vi "rsidr_core_global.vi"() -> ()   [LabVIEW 2015, in "Rohde&Schwarz CMXP GPRF.lvlib"]
doc: "This Global variable contains driver's:\n- Attributes\n- Range Tables\n- Repeated Capabilities"
uses:
  <instrlib>/Rohde&Schwarz CMXP GPRF/Rohde&Schwarz CMXP GPRF.lvlib
  <instrlib>/Rohde&Schwarz CMXP GPRF/Private/rsidr_core.llb/type_Input_Format_Attribute.ctl
  <instrlib>/Rohde&Schwarz CMXP GPRF/Private/rsidr_core.llb/type_Input_Format_RangeTable.ctl
  <instrlib>/Rohde&Schwarz CMXP GPRF/Private/rsidr_core.llb/type_Input_Format_RepCap.ctl
  <instrlib>/Rohde&Schwarz CMXP GPRF/Private/rsidr_core.llb/rsidr_core.lvlib
panel:
  in  "Repeated Capabilities":T1[](array[typedef])
  in  "Range Tables":T2[](array[typedef])=[{"Type"=2, "Name"="rsCmxpGprf_rngInputConnector", "Entries"=[{"Name"="RF 1 COM", "Value 1"=1.0, "Value 2"=0.0, "Command"="RF1C"}, {"Name"="RF 2 COM", "Value 1"=2.0, "Value 2"=0.0, "Command"="RF2C"}, {"Name"="RF 2 IN", "Value 1"=3.0, "Value 2"=0.0, "Command"="RF2I"}, {"Name"="RF 3 COM", "Value 1"=4.0, "Value 2"=0.0, "Command"="RF3C"}, {"Name"="RF 4 COM", "Value 1"=5.0, "Value 2"=0.0, "Command"="RF4C"}, {"Name"="RF 4 IN", "Value 1"=6.0, "Value 2"=0.0, "Command"="RF4I"}, {"Name"="IQ 1 IN", "Value 1"=7.0, "Value 2"=0.0, "Command"="IQ1I"}, {"Name"="IQ 3 IN", "Value 1"=8.0, "Value 2"=0.0, "Command"="IQ3I"}, {"Name"="IQ 5 IN", "Value 1"=9.0, "Value 2"=0.0, "Command"="IQ5I"}, {"Name"="IQ 7 IN", "Value 1"=10.0, "Value 2"=0.0, "Command"="IQ7I"}, {"Name"="RF 11", "Value 1"=11.0, "Value 2"=0.0, "Command"="R11"}, {"Name"="RF 12", "Value 1"=12.0, "Value 2"=0.0, "Command"="R12"}, {"Name"="RF 13", "Value 1"=13.0, "Value 2"=0.0, "Command"="R13"}, {"Name"="RF 14", "Value 1"=14.0, "Value 2"=0.0, "Command"="R14"}, {"Name"="RF 15", "Value 1"=15.0, "Value 2"=0.0, "Command"="R15"}, {"Name"="RF 16", "Value 1"=16.0, "Value 2"=0.0, "Command"="R16"}, {"Name"="RF 17", "Value 1"=17.0, "Value 2"=0.0, "Command"="R17"}, {"Name"="RF 18", "Value 1"=18.0, "Value 2"=0.0, "Command"="R18"}, {"Name"="RF 21", "Value 1"=19.0, "Value 2"=0.0, "Command"="R21"}, {"Name"="RF 22", "Value 1"=20.0, "Value 2"=0.0, "Command"="R22"}, {"Name"="RF 23", "Value 1"=21.0, "Value 2"=0.0, "Command"="R23"}, {"Name"="RF 24", "Value 1"=22.0, "Value 2"=0.0, "Command"="R24"}, {"Name"="RF 25", "Value 1"=23.0, "Value 2"=0.0, "Command"="R25"}, {"Name"="RF 26", "Value 1"=24.0, "Value 2"=0.0, "Command"="R26"}, {"Name"="RF 27", "Value 1"=25.0, "Value 2"=0.0, "Command"="R27"}, {"Name"="RF 28", "Value 1"=26.0, "Value 2"=0.0, "Command"="R28"}, {"Name"="RF 31", "Value 1"=27.0, "Value 2"=0.0, "Command"="R31"}, {"Name"="RF 32", "Value 1"=28.0, "Value 2"=0.0, "Command"="R32"}, {"Name"="RF 33", "Value 1"=29.0, "Value 2"=0.0, "Command"="R33"}, {"Name"="RF 34", "Value 1"=30.0, "Value 2"=0.0, "Command"="R34"}, {"Name"="RF 35", "Value 1"=31.0, "Value 2"=0.0, "Command"="R35"}, {"Name"="RF 36", "Value 1"=32.0, "Value 2"=0.0, "Command"="R36"}, {"Name"="RF 37", "Value 1"=33.0, "Value 2"=0.0, "Command"="R37"}, {"Name"="RF 38", "Value 1"=34.0, "Value 2"=0.0, "Command"="R38"}, {"Name"="RF 41", "Value 1"=35.0, "Value 2"=0.0, "Command"="R41"}, {"Name"="RF 42", "Value 1"=36.0, "Value 2"=0.0, "Command"="R42"}, {"Name"="RF 43", "Value 1"=37.0, "Value 2"=0.0, "Command"="R43"}, {"Name"="RF 44", "Value 1"=38.0, "Value 2"=0.0, "Command"="R44"}, {"Name"="RF 45", "Value 1"=39.0, "Value 2"=0.0, "Command"="R45"}, {"Name"="RF 46", "Value 1"=40.0, "Value 2"=0.0, "Command"="R46"}, {"Name"="RF 47", "Value 1"=41.0, "Value 2"=0.0, "Command"="R47"}, {"Name"="RF 48", "Value 1"=42.0, "Value 2"=0.0, "Command"="R48"}, {"Name"="RF 11 COM", "Value 1"=43.0, "Value 2"=0.0, "Command"="R11C"}, {"Name"="RF 12 COM", "Value 1"=44.0, "Value 2"=0.0, "Command"="R12C"}, {"Name"="RF 12 IN", "Value 1"=45.0, "Value 2"=0.0, "Command"="R12I"}, {"Name"="RF 13 COM", "Value 1"=46.0, "Value 2"=0.0, "Command"="R13C"}, {"Name"="RF 14 COM", "Value 1"=47.0, "Value 2"=0.0, "Command"="R14C"}, {"Name"="RF 14 IN", "Value 1"=48.0, "Value 2"=0.0, "Command"="R14I"}, {"Name"="IQ 11 IN", "Value 1"=49.0, "Value 2"=0.0, "Command"="I11I"}, {"Name"="IQ 13 IN", "Value 1"=50.0, "Value 2"=0.0, "Command"="I13I"}, {"Name"="IQ 15 IN", "Value 1"=51.0, "Value 2"=0.0, "Command"="I15I"}, {"Name"="IQ 17 IN", "Value 1"=52.0, "Value 2"=0.0, "Command"="I17I"}, {"Name"="RF 21 COM", "Value 1"=53.0, "Value 2"=0.0, "Command"="R21C"}, {"Name"="RF 22 COM", "Value 1"=54.0, "Value 2"=0.0, "Command"="R22C"}, {"Name"="RF 22 IN", "Value 1"=55.0, "Value 2"=0.0, "Command"="R22I"}, {"Name"="RF 23 COM", "Value 1"=56.0, "Value 2"=0.0, "Command"="R23C"}, {"Name"="RF 24 COM", "Value 1"=57.0, "Value 2"=0.0, "Command"="R24C"}, {"Name"="RF 24 IN", "Value 1"=58.0, "Value 2"=0.0, "Command"="R24I"}, {"Name"="IQ 21 IN", "Value 1"=59.0, "Value 2"=0.0, "Command"="I21I"}, {"Name"="IQ 23 IN", "Value 1"=60.0, "Value 2"=0.0, "Command"="I23I"}, {"Name"="IQ 25 IN", "Value 1"=61.0, "Value 2"=0.0, "Command"="I25I"}, {"Name"="IQ 27 IN", "Value 1"=62.0, "Value 2"=0.0, "Command"="I27I"}, {"Name"="RF 31 COM", "Value 1"=63.0, "Value 2"=0.0, "Command"="R31C"}, {"Name"="RF 32 COM", "Value 1"=64.0, "Value 2"=0.0, "Command"="R32C"}, {"Name"="RF 32 IN", "Value 1"=65.0, "Value 2"=0.0, "Command"="R32I"}, {"Name"="RF 33 COM", "Value 1"=66.0, "Value 2"=0.0, "Command"="R33C"}, {"Name"="RF 34 COM", "Value 1"=67.0, "Value 2"=0.0, "Command"="R34C"}, {"Name"="RF 34 IN", "Value 1"=68.0, "Value 2"=0.0, "Command"="R34I"}, {"Name"="IQ 31 IN", "Value 1"=69.0, "Value 2"=0.0, "Command"="I31I"}, {"Name"="IQ 33 IN", "Value 1"=70.0, "Value 2"=0.0, "Command"="I33I"}, {"Name"="IQ 35 IN", "Value 1"=71.0, "Value 2"=0.0, "Command"="I35I"}, {"Name"="IQ 37 IN", "Value 1"=72.0, "Value 2"=0.0, "Command"="I37I"}, {"Name"="RF 41 COM", "Value 1"=73.0, "Value 2"=0.0, "Command"="R41C"}, {"Name"="RF 42 COM", "Value 1"=74.0, "Value 2"=0.0, "Command"="R42C"}, {"Name"="RF 42 IN", "Value 1"=75.0, "Value 2"=0.0, "Command"="R42I"}, {"Name"="RF 43 COM", "Value 1"=76.0, "Value 2"=0.0, "Command"="R43C"}, {"Name"="RF 44 COM", "Value 1"=77.0, "Value 2"=0.0, "Command"="R44C"}, {"Name"="RF 44 IN", "Value 1"=78.0, "Value 2"=0.0, "Command"="R44I"}, {"Name"="IQ 41 IN", "Value 1"=79.0, "Value 2"=0.0, "Command"="I41I"}, {"Name"="IQ 43 IN", "Value 1"=80.0, "Value 2"=0.0, "Command"="I43I"}, {"Name"="IQ 45 IN", "Value 1"=81.0, "Value 2"=0.0, "Command"="I45I"}, {"Name"="IQ 47 IN", "Value 1"=82.0, "Value 2"=0.0, "Command"="I47I"}, {"Name"="RF A COM", "Value 1"=83.0, "Value 2"=0.0, "Command"="RFAC"}, {"Name"="RF B COM", "Value 1"=84.0, "Value 2"=0.0, "Command"="RFBC"}, {"Name"="RF B IN", "Value 1"=85.0, "Value 2"=0.0, "Command"="RFBI"}, {"Name"="RF A 1", "Value 1"=86.0, "Value 2"=0.0, "Command"="RA1"}, {"Name"="RF A 2", "Value 1"=87.0, "Value 2"=0.0, "Command"="RA2"}, {"Name"="RF A 3", "Value 1"=88.0, "Value 2"=0.0, "Command"="RA3"}, {"Name"="RF A 4", "Value 1"=89.0, "Value 2"=0.0, "Command"="RA4"}, {"Name"="RF A 5", "Value 1"=90.0, "Value 2"=0.0, "Command"="RA5"}, {"Name"="RF A 6", "Value 1"=91.0, "Value 2"=0.0, "Command"="RA6"}, {"Name"="RF A 7", "Value 1"=92.0, "Value 2"=0.0, "Command"="RA7"}, {"Name"="RF A 8", "Value 1"=93.0, "Value 2"=0.0, "Command"="RA8"}, {"Name"="RF B 1", "Value 1"=94.0, "Value 2"=0.0, "Command"="RB1"}, {"Name"="RF B 2", "Value 1"=95.0, "Value 2"=0.0, "Command"="RB2"}, {"Name"="RF B 3", "Value 1"=96.0, "Value 2"=0.0, "Command"="RB3"}, {"Name"="RF B 4", "Value 1"=97.0, "Value 2"=0.0, "Command"="RB4"}, {"Name"="RF B 5", "Value 1"=98.0, "Value 2"=0.0, "Command"="RB5"}, {"Name"="RF B 6", "Value 1"=99.0, "Value 2"=0.0, "Command"="RB6"}, {"Name"="RF B 7", "Value 1"=100.0, "Value 2"=0.0, "Command"="RB7"}, {"Name"="RF B 8", "Value 1"=101.0, "Value 2"=0.0, "Command"="RB8"}]}, {"Type"=0, "Name"="rsCmxpGprf_rngExtAtt", "Entries"=[{"Name"="", "Value 1"=-50.0, "Value 2"=90.0, "Command"=""}]}, {"Type"=0, "Name"="rsCmxpGprf_rngCenterFrequency", "Entries"=[{"Name"="", "Value 1"=70000000.0, "Value 2"=6000000000.0, "Command"=""}]}, {"Type"=2, "Name"="rsCmxpGprf_rngOutputConnector", "Entries"=[{"Name"="RF 1 OUT", "Value 1"=0.0, "Value 2"=0.0, "Command"="RF1O"}, {"Name"="RF 1 COM", "Value 1"=1.0, "Value 2"=0.0, "Command"="RF1C"}, {"Name"="RF 2 COM", "Value 1"=2.0, "Value 2"=0.0, "Command"="RF2C"}, {"Name"="RF 3 COM", "Value 1"=3.0, "Value 2"=0.0, "Command"="RF3C"}, {"Name"="RF 3 OUT", "Value 1"=4.0, "Value 2"=0.0, "Command"="RF3O"}, {"Name"="RF 4 COM", "Value 1"=5.0, "Value 2"=0.0, "Command"="RF4C"}, {"Name"="IQ 2 OUT", "Value 1"=6.0, "Value 2"=0.0, "Command"="IQ2O"}, {"Name"="IQ 4 OUT", "Value 1"=7.0, "Value 2"=0.0, "Command"="IQ4O"}, {"Name"="IQ 6 OUT", "Value 1"=8.0, "Value 2"=0.0, "Command"="IQ6O"}, {"Name"="IQ 8 OUT", "Value 1"=9.0, "Value 2"=0.0, "Command"="IQ8O"}, {"Name"="RF 118", "Value 1"=10.0, "Value 2"=0.0, "Command"="R118"}, {"Name"="RF 218", "Value 1"=11.0, "Value 2"=0.0, "Command"="R218"}, {"Name"="RF 214", "Value 1"=12.0, "Value 2"=0.0, "Command"="R214"}, {"Name"="RF 258", "Value 1"=13.0, "Value 2"=0.0, "Command"="R258"}, {"Name"="RF 318", "Value 1"=14.0, "Value 2"=0.0, "Command"="R318"}, {"Name"="RF 418", "Value 1"=15.0, "Value 2"=0.0, "Command"="R418"}, {"Name"="RF 11 COM", "Value 1"=16.0, "Value 2"=0.0, "Command"="R11C"}, {"Name"="RF 11 OUT", "Value 1"=17.0, "Value 2"=0.0, "Command"="R11O"}, {"Name"="RF 12 COM", "Value 1"=18.0, "Value 2"=0.0, "Command"="R12C"}, {"Name"="RF 13 COM", "Value 1"=19.0, "Value 2"=0.0, "Command"="R13C"}, {"Name"="RF 13 OUT", "Value 1"=20.0, "Value 2"=0.0, "Command"="R13O"}, {"Name"="RF 14 COM", "Value 1"=21.0, "Value 2"=0.0, "Command"="R14C"}, {"Name"="IQ 12 OUT", "Value 1"=22.0, "Value 2"=0.0, "Command"="I12O"}, {"Name"="IQ 14 OUT", "Value 1"=23.0, "Value 2"=0.0, "Command"="I14O"}, {"Name"="IQ 16 OUT", "Value 1"=24.0, "Value 2"=0.0, "Command"="I16O"}, {"Name"="IQ 18 OUT", "Value 1"=25.0, "Value 2"=0.0, "Command"="I18O"}, {"Name"="RF 21 COM", "Value 1"=26.0, "Value 2"=0.0, "Command"="R21C"}, {"Name"="RF 21 OUT", "Value 1"=27.0, "Value 2"=0.0, "Command"="R21O"}, {"Name"="RF 22 COM", "Value 1"=28.0, "Value 2"=0.0, "Command"="R22C"}, {"Name"="RF 23 COM", "Value 1"=29.0, "Value 2"=0.0, "Command"="R23C"}, {"Name"="RF 23 OUT", "Value 1"=30.0, "Value 2"=0.0, "Command"="R23O"}, {"Name"="RF 24 COM", "Value 1"=31.0, "Value 2"=0.0, "Command"="R24C"}, {"Name"="IQ 22 OUT", "Value 1"=32.0, "Value 2"=0.0, "Command"="I22O"}, {"Name"="IQ 24 OUT", "Value 1"=33.0, "Value 2"=0.0, "Command"="I24O"}, {"Name"="IQ 26 OUT", "Value 1"=34.0, "Value 2"=0.0, "Command"="I26O"}, {"Name"="IQ 28 OUT", "Value 1"=35.0, "Value 2"=0.0, "Command"="I28O"}, {"Name"="RF 31 COM", "Value 1"=36.0, "Value 2"=0.0, "Command"="R31C"}, {"Name"="RF 31 OUT", "Value 1"=37.0, "Value 2"=0.0, "Command"="R31O"}, {"Name"="RF 32 COM", "Value 1"=38.0, "Value 2"=0.0, "Command"="R32C"}, {"Name"="RF 33 COM", "Value 1"=39.0, "Value 2"=0.0, "Command"="R33C"}, {"Name"="RF 33 OUT", "Value 1"=40.0, "Value 2"=0.0, "Command"="R33O"}, {"Name"="RF 34 COM", "Value 1"=41.0, "Value 2"=0.0, "Command"="R34C"}, {"Name"="IQ 32 OUT", "Value 1"=42.0, "Value 2"=0.0, "Command"="I32O"}, {"Name"="IQ 34 OUT", "Value 1"=43.0, "Value 2"=0.0, "Command"="I34O"}, {"Name"="IQ 36 OUT", "Value 1"=44.0, "Value 2"=0.0, "Command"="I36O"}, {"Name"="IQ 38 OUT", "Value 1"=45.0, "Value 2"=0.0, "Command"="I38O"}, {"Name"="RF 41 COM", "Value 1"=46.0, "Value 2"=0.0, "Command"="R41C"}, {"Name"="RF 41 OUT", "Value 1"=47.0, "Value 2"=0.0, "Command"="R41O"}, {"Name"="RF 42 COM", "Value 1"=48.0, "Value 2"=0.0, "Command"="R42C"}, {"Name"="RF 43 COM", "Value 1"=49.0, "Value 2"=0.0, "Command"="R43C"}, {"Name"="RF 43 OUT", "Value 1"=50.0, "Value 2"=0.0, "Command"="R43O"}, {"Name"="RF 44 COM", "Value 1"=51.0, "Value 2"=0.0, "Command"="R44C"}, {"Name"="IQ 42 OUT", "Value 1"=52.0, "Value 2"=0.0, "Command"="I42O"}, {"Name"="IQ 44 OUT", "Value 1"=53.0, "Value 2"=0.0, "Command"="I44O"}, {"Name"="IQ 46 OUT", "Value 1"=54.0, "Value 2"=0.0, "Command"="I46O"}, {"Name"="IQ 48 OUT", "Value 1"=55.0, "Value 2"=0.0, "Command"="I48O"}, {"Name"="RF A COM", "Value 1"=56.0, "Value 2"=0.0, "Command"="RFAC"}, {"Name"="RF A OUT", "Value 1"=57.0, "Value 2"=0.0, "Command"="RFAO"}, {"Name"="RF B COM", "Value 1"=58.0, "Value 2"=0.0, "Command"="RFBC"}, {"Name"="RF A 18", "Value 1"=59.0, "Value 2"=0.0, "Command"="RA18"}, {"Name"="RF B 14", "Value 1"=60.0, "Value 2"=0.0, "Command"="RB14"}, {"Name"="RF B 18", "Value 1"=61.0, "Value 2"=0.0, "Command"="RB18"}]}, {"Type"=0, "Name"="rsCmxpGprf_rngGeneratorLevel", "Entries"=[{"Name"="", "Value 1"=-130.0, "Value 2"=0.0, "Command"=""}]}, {"Type"=2, "Name"="rsCmxpGprf_rngBasebandMode", "Entries"=[{"Name"="CW", "Value 1"=0.0, "Value 2"=0.0, "Command"="CW"}, {"Name"="Dual Tone", "Value 1"=1.0, "Value 2"=0.0, "Command"="DTON"}, {"Name"="ARB", "Value 1"=2.0, "Value 2"=0.0, "Command"="ARB"}]}, {"Type"=0, "Name"="rsCmxpGprf_rngDtoneFrequency", "Entries"=[{"Name"="", "Value 1"=-40000000.0, "Value 2"=40000000.0, "Command"=""}]}, {"Type"=0, "Name"="rsCmxpGprf_rngDtoneRatio", "Entries"=[{"Name"="", "Value 1"=0.0, "Value 2"=30.0, "Command"=""}]}, {"Type"=0, "Name"="rsCmxpGprf_rngListModeDwellTime", "Entries"=[{"Name"="", "Value 1"=0.0002, "Value 2"=20.0, "Command"=""}]}, {"Type"=0, "Name"="rsCmxpGprf_rngListLevel", "Entries"=[{"Name"="", "Value 1"=-130.0, "Value 2"=13.0, "Command"=""}]}, {"Type"=0, "Name"="rsCmxpGprf_rngDigitalGain", "Entries"=[{"Name"="", "Value 1"=-30.0, "Value 2"=0.0, "Command"=""}]}, {"Type"=0, "Name"="rsCmxpGprf_rngStepLength", "Entries"=[{"Name"="", "Value 1"=5e-05, "Value 2"=1.0, "Command"=""}]}, {"Type"=0, "Name"="rsCmxpGprf_rngMeasLength", "Entries"=[{"Name"="", "Value 1"=5e-05, "Value 2"=0.0003, "Command"=""}]}, {"Type"=2, "Name"="rsCmxpGprf_rngRepMode", "Entries"=[{"Name"="Single", "Value 1"=0.0, "Value 2"=0.0, "Command"="SING"}, {"Name"="Continuous", "Value 1"=1.0, "Value 2"=0.0, "Command"="CONT"}]}, {"Type"=0, "Name"="rsCmxpGprf_rngStatCount", "Entries"=[{"Name"="", "Value 1"=1.0, "Value 2"=1000.0, "Command"=""}]}, {"Type"=2, "Name"="rsCmxpGprf_rngPowerMeasFilterType", "Entries"=[{"Name"="Gauss", "Value 1"=0.0, "Value 2"=0.0, "Command"="GAUS"}, {"Name"="Bandpass", "Value 1"=1.0, "Value 2"=0.0, "Command"="BAND"}, {"Name"="WCDMA", "Value 1"=2.0, "Value 2"=0.0, "Command"="WCDM"}, {"Name"="CDMA", "Value 1"=3.0, "Value 2"=0.0, "Command"="CDMA"}, {"Name"="TD-SCDMA", "Value 1"=4.0, "Value 2"=0.0, "Command"="TDSC"}]}, {"Type"=1, "Name"="rsCmxpGprf_rngGaussBwid", "Entries"=[{"Name"="", "Value 1"=1000.0, "Value 2"=0.0, "Command"=""}, {"Name"="", "Value 1"=10000.0, "Value 2"=0.0, "Command"=""}, {"Name"="", "Value 1"=100000.0, "Value 2"=0.0, "Command"=""}, {"Name"="", "Value 1"=1000000.0, "Value 2"=0.0, "Command"=""}, {"Name"="", "Value 1"=10000000.0, "Value 2"=0.0, "Command"=""}]}, {"Type"=1, "Name"="rsCmxpGprf_rngBandBwid", "Entries"=[{"Name"="", "Value 1"=1000.0, "Value 2"=0.0, "Command"=""}, {"Name"="", "Value 1"=10000.0, "Value 2"=0.0, "Command"=""}, {"Name"="", "Value 1"=100000.0, "Value 2"=0.0, "Command"=""}, {"Name"="", "Value 1"=1000000.0, "Value 2"=0.0, "Command"=""}, {"Name"="", "Value 1"=10000000.0, "Value 2"=0.0, "Command"=""}, {"Name"="", "Value 1"=40000000.0, "Value 2"=0.0, "Command"=""}, {"Name"="", "Value 1"=160000000.0, "Value 2"=0.0, "Command"=""}]}, {"Type"=2, "Name"="rsCmxpGprf_rngTrigSlope", "Entries"=[{"Name"="Rising", "Value 1"=0.0, "Value 2"=0.0, "Command"="REDG"}, {"Name"="Falling", "Value 1"=1.0, "Value 2"=0.0, "Command"="FEDG"}]}, {"Type"=0, "Name"="rsCmxpGprf_rngTrigThreshold", "Entries"=[{"Name"="", "Value 1"=-50.0, "Value 2"=0.0, "Command"=""}]}, {"Type"=0, "Name"="rsCmxpGprf_rngTrigOffset", "Entries"=[{"Name"="", "Value 1"=-0.15, "Value 2"=0.15, "Command"=""}]}, {"Type"=0, "Name"="rsCmxpGprf_rngTrigTout", "Entries"=[{"Name"="", "Value 1"=0.01, "Value 2"=300.0, "Command"=""}]}, {"Type"=2, "Name"="rsCmxpGprf_rngTrigMode", "Entries"=[{"Name"="Trigger Once", "Value 1"=0.0, "Value 2"=0.0, "Command"="ONCE"}, {"Name"="Retrigger Sweep", "Value 1"=1.0, "Value 2"=0.0, "Command"="SWE"}, {"Name"="Retrigger All", "Value 1"=2.0, "Value 2"=0.0, "Command"="ALL"}, {"Name"="Preselect", "Value 1"=3.0, "Value 2"=0.0, "Command"="PRES"}]}, {"Type"=0, "Name"="rsCmxpGprf_rngPwrListIndex", "Entries"=[{"Name"="", "Value 1"=0.0, "Value 2"=3999.0, "Command"=""}]}, {"Type"=2, "Name"="rsCmxpGprf_rngResolution", "Entries"=[{"Name"="1 dB", "Value 1"=0.0, "Value 2"=0.0, "Command"="PD0"}, {"Name"="0.1 dB", "Value 1"=1.0, "Value 2"=0.0, "Command"="PD1"}, {"Name"="0.01 dB", "Value 1"=2.0, "Value 2"=0.0, "Command"="PD2"}, {"Name"="0.001 dB", "Value 1"=3.0, "Value 2"=0.0, "Command"="PD3"}]}, {"Type"=0, "Name"="rsCmxpGprf_rngExtSensorAttenuation", "Entries"=[{"Name"="", "Value 1"=-50.0, "Value 2"=50.0, "Command"=""}]}, {"Type"=0, "Name"="rsCmxpGprf_rngIqvsStepLength", "Entries"=[{"Name"="", "Value 1"=5e-05, "Value 2"=0.005, "Command"=""}]}, {"Type"=0, "Name"="rsCmxpGprf_rngIqvsMeasLength", "Entries"=[{"Name"="", "Value 1"=1e-05, "Value 2"=0.001, "Command"=""}]}, {"Type"=0, "Name"="rsCmxpGprf_rngIqvsFELimit", "Entries"=[{"Name"="", "Value 1"=-100.0, "Value 2"=-30.0, "Command"=""}]}, {"Type"=0, "Name"="rsCmxpGprf_rngIqvsCount", "Entries"=[{"Name"="", "Value 1"=1.0, "Value 2"=3000.0, "Command"=""}]}, {"Type"=2, "Name"="rsCmxpGprf_rngIqvsFilterType", "Entries"=[{"Name"="Gauss", "Value 1"=0.0, "Value 2"=0.0, "Command"="GAUS"}, {"Name"="Bandpass 1MHz", "Value 1"=1.0, "Value 2"=0.0, "Command"="B1MH"}, {"Name"="Nyquist 1MHz", "Value 1"=2.0, "Value 2"=0.0, "Command"="NY1M"}, {"Name"="Bandpass 10MHz", "Value 1"=3.0, "Value 2"=0.0, "Command"="B10M"}, {"Name"="Nyquist 100kHz", "Value 1"=4.0, "Value 2"=0.0, "Command"="NYQ"}]}, {"Type"=0, "Name"="rsCmxpGprf_rngTriggerGap", "Entries"=[{"Name"="", "Value 1"=0.0, "Value 2"=0.01, "Command"=""}]}, {"Type"=0, "Name"="rsCmxpGprf_rngIqvsListIndex", "Entries"=[{"Name"="", "Value 1"=0.0, "Value 2"=149.0, "Command"=""}]}, {"Type"=2, "Name"="rsCmxpGprf_rngIqRFilterType", "Entries"=[{"Name"="Gauss", "Value 1"=0.0, "Value 2"=0.0, "Command"="GAUS"}, {"Name"="Bandpass", "Value 1"=1.0, "Value 2"=0.0, "Command"="BAND"}]}, {"Type"=1, "Name"="rsCmxpGprf_rngFFTFrequencySpan", "Entries"=[{"Name"="", "Value 1"=1250000.0, "Value 2"=0.0, "Command"=""}, {"Name"="", "Value 1"=2500000.0, "Value 2"=0.0, "Command"=""}, {"Name"="", "Value 1"=5000000.0, "Value 2"=0.0, "Command"=""}, {"Name"="", "Value 1"=10000000.0, "Value 2"=0.0, "Command"=""}, {"Name"="", "Value 1"=20000000.0, "Value 2"=0.0, "Command"=""}, {"Name"="", "Value 1"=40000000.0, "Value 2"=0.0, "Command"=""}]}, {"Type"=1, "Name"="rsCmxpGprf_rngFFTLength", "Entries"=[{"Name"="", "Value 1"=1024.0, "Value 2"=0.0, "Command"=""}, {"Name"="", "Value 1"=2048.0, "Value 2"=0.0, "Command"=""}, {"Name"="", "Value 1"=4096.0, "Value 2"=0.0, "Command"=""}, {"Name"="", "Value 1"=8192.0, "Value 2"=0.0, "Command"=""}, {"Name"="", "Value 1"=16384.0, "Value 2"=0.0, "Command"=""}]}, {"Type"=2, "Name"="rsCmxpGprf_rngFFTDetector", "Entries"=[{"Name"="Peak", "Value 1"=0.0, "Value 2"=0.0, "Command"="PEAK"}, {"Name"="RMS", "Value 1"=1.0, "Value 2"=0.0, "Command"="RMS"}]}, {"Type"=0, "Name"="rsCmxpGprf_rngARBCycles", "Entries"=[{"Name"="", "Value 1"=1.0, "Value 2"=10000.0, "Command"=""}]}, {"Type"=2, "Name"="rsCmxpGprf_rngARBMultisegmentTriggerMode", "Entries"=[{"Name"="Seamless", "Value 1"=0.0, "Value 2"=0.0, "Command"="CSE"}, {"Name"="Continuous", "Value 1"=1.0, "Value 2"=0.0, "Command"="CONT"}, {"Name"="Auto", "Value 1"=2.0, "Value 2"=0.0, "Command"="AUTO"}]}, {"Type"=0, "Name"="rsCmxpGprf_rngIndex", "Entries"=[{"Name"="", "Value 1"=0.0, "Value 2"=1999.0, "Command"=""}]}, {"Type"=0, "Name"="rsCmxpGprf_rngIQvsSlotRatio", "Entries"=[{"Name"="", "Value 1"=0.1, "Value 2"=1.0, "Command"=""}]}, {"Type"=0, "Name"="rsCmxpGprf_rngPeakSearchMarkers", "Entries"=[{"Name"="", "Value 1"=0.0, "Value 2"=5.0, "Command"=""}]}, {"Type"=2, "Name"="rsCmxpGprf_rngLinLog", "Entries"=[{"Name"="Linear", "Value 1"=0.0, "Value 2"=0.0, "Command"="LIN"}, {"Name"="Logarithmic", "Value 1"=1.0, "Value 2"=0.0, "Command"="LOG"}]}, {"Type"=2, "Name"="rsCmxpGprf_rngScenario", "Entries"=[{"Name"="Standalone", "Value 1"=0.0, "Value 2"=0.0, "Command"="STAN"}, {"Name"="Combined Signal Path", "Value 1"=1.0, "Value 2"=0.0, "Command"="CSP"}]}, {"Type"=2, "Name"="rsCmxpGprf_rngFFTTriggerOffsetMode", "Entries"=[{"Name"="Fixed", "Value 1"=0.0, "Value 2"=0.0, "Command"="FIX"}, {"Name"="Variable", "Value 1"=1.0, "Value 2"=0.0, "Command"="VAR"}]}, {"Type"=0, "Name"="rsCmxpGprf_rngTrigOffsetIFPow", "Entries"=[{"Name"="", "Value 1"=0.0, "Value 2"=1.0, "Command"=""}]}, {"Type"=2, "Name"="rsCmxpGprf_rngGeneratorState", "Entries"=[{"Name"="Off", "Value 1"=0.0, "Value 2"=0.0, "Command"="OFF"}, {"Name"="On", "Value 1"=1.0, "Value 2"=0.0, "Command"="ON"}, {"Name"="Pending", "Value 1"=2.0, "Value 2"=0.0, "Command"="PEND"}, {"Name"="Adjusted", "Value 1"=3.0, "Value 2"=0.0, "Command"="ADJ"}, {"Name"="Autonomous", "Value 1"=4.0, "Value 2"=0.0, "Command"="AUT"}, {"Name"="Coupled", "Value 1"=5.0, "Value 2"=0.0, "Command"="COUP"}, {"Name"="Invalid", "Value 1"=6.0, "Value 2"=0.0, "Command"="INV"}]}, {"Type"=2, "Name"="rsCmxpGprf_rngIQvsSlotTriggMode", "Entries"=[{"Name"="Once", "Value 1"=0.0, "Value 2"=0.0, "Command"="ONCE"}, {"Name"="Preselect", "Value 1"=1.0, "Value 2"=0.0, "Command"="PRES"}]}, {"Type"=2, "Name"="rsCmxpGprf_rngPwrMeasParameterSet", "Entries"=[{"Name"="Global", "Value 1"=0.0, "Value 2"=0.0, "Command"="GLOB"}, {"Name"="Independent", "Value 1"=1.0, "Value 2"=0.0, "Command"="LIST"}]}, {"Type"=2, "Name"="rsCmxpGprf_rngIQRecorderMeasMagnitudeUnit", "Entries"=[{"Name"="Voltage unit", "Value 1"=0.0, "Value 2"=0.0, "Command"="VOLT"}, {"Name"="Raw I/Q data", "Value 1"=1.0, "Value 2"=0.0, "Command"="RAW"}]}, {"Type"=1, "Name"="rsCmxpGprf_rngDigitalIQSampleRate", "Entries"=[{"Name"="", "Value 1"=1920000.0, "Value 2"=0.0, "Command"=""}, {"Name"="", "Value 1"=3840000.0, "Value 2"=0.0, "Command"=""}, {"Name"="", "Value 1"=7680000.0, "Value 2"=0.0, "Command"=""}, {"Name"="", "Value 1"=9600000.0, "Value 2"=0.0, "Command"=""}, {"Name"="", "Value 1"=15360000.0, "Value 2"=0.0, "Command"=""}, {"Name"="", "Value 1"=19200000.0, "Value 2"=0.0, "Command"=""}, {"Name"="", "Value 1"=30720000.0, "Value 2"=0.0, "Command"=""}, {"Name"="", "Value 1"=100000000.0, "Value 2"=0.0, "Command"=""}]}, {"Type"=2, "Name"="rsCmxpGprf_rngDigitalIQTransferMode", "Entries"=[{"Name"="Enable Mode", "Value 1"=0.0, "Value 2"=0.0, "Command"="ENAB"}, {"Name"="Request Mode", "Value 1"=1.0, "Value 2"=0.0, "Command"="REQ"}]}, {"Type"=0, "Name"="rsCmxpGprf_rngARBFrequencyOffset", "Entries"=[{"Name"="", "Value 1"=-40000000.0, "Value 2"=40000000.0, "Command"=""}]}, {"Type"=0, "Name"="rsCmxpGprf_rngARBTriggerDelay", "Entries"=[{"Name"="", "Value 1"=0.0, "Value 2"=100.0, "Command"=""}]}, {"Type"=2, "Name"="rsCmxpGprf_rngNoYesNav", "Entries"=[{"Name"="No", "Value 1"=0.0, "Value 2"=0.0, "Command"="NO"}, {"Name"="Yes", "Value 1"=1.0, "Value 2"=0.0, "Command"="YES"}, {"Name"="Not a value", "Value 1"=-1.0, "Value 2"=0.0, "Command"="NAV"}]}, {"Type"=2, "Name"="rsCmxpGprf_rngARBFileCRCProtection", "Entries"=[{"Name"="No", "Value 1"=0.0, "Value 2"=0.0, "Command"="NO"}, {"Name"="Yes", "Value 1"=1.0, "Value 2"=0.0, "Command"="YES"}, {"Name"="Not a value", "Value 1"=-1.0, "Value 2"=0.0, "Command"="NAV"}]}, {"Type"=2, "Name"="rsCmxpGprf_rngPowerMeasurementResultMode", "Entries"=[{"Name"="Power", "Value 1"=0.0, "Value 2"=0.0, "Command"="POW"}, {"Name"="Statistic", "Value 1"=1.0, "Value 2"=0.0, "Command"="STAT"}]}, {"Type"=0, "Name"="rsCmxpGprf_rngSpecFreq", "Entries"=[{"Name"="", "Value 1"=70000000.0, "Value 2"=6000000000.0, "Command"=""}]}, {"Type"=2, "Name"="rsCmxpGprf_rngIQRecMeasFormat", "Entries"=[{"Name"="Cartesian Coordinates", "Value 1"=0.0, "Value 2"=0.0, "Command"="IQ"}, {"Name"="Polar Coordinates", "Value 1"=1.0, "Value 2"=0.0, "Command"="RPHI"}]}, {"Type"=2, "Name"="rsCmxpGprf_rngPowerMeasurementTriggerTXIncrementTiming", "Entries"=[{"Name"="Step", "Value 1"=0.0, "Value 2"=0.0, "Command"="STEP"}, {"Name"="Centered", "Value 1"=1.0, "Value 2"=0.0, "Command"="CENT"}]}, {"Type"=2, "Name"="rsCmxpGprf_rngPowerMeasTXIncrement", "Entries"=[{"Name"="Step", "Value 1"=0.0, "Value 2"=0.0, "Command"="STEP"}, {"Name"="Center", "Value 1"=1.0, "Value 2"=0.0, "Command"="CENT"}]}, {"Type"=0, "Name"="rsCmxpGprf_rngPwrListStart", "Entries"=[{"Name"="", "Value 1"=0.0, "Value 2"=1999.0, "Command"=""}]}, {"Type"=2, "Name"="rsCmxpGprf_rngIQRecorderWriteResultToIQFile", "Entries"=[{"Name"="Off", "Value 1"=0.0, "Value 2"=0.0, "Command"="OFF"}, {"Name"="On", "Value 1"=1.0, "Value 2"=0.0, "Command"="ON"}, {"Name"="Only", "Value 1"=2.0, "Value 2"=0.0, "Command"="ONLY"}]}, {"Type"=1, "Name"="rsCmxpGprf_rngPowerBandpassBandwidth", "Entries"=[{"Name"="", "Value 1"=1000.0, "Value 2"=0.0, "Command"=""}, {"Name"="", "Value 1"=3000.0, "Value 2"=0.0, "Command"=""}, {"Name"="", "Value 1"=5000.0, "Value 2"=0.0, "Command"=""}, {"Name"="", "Value 1"=10000.0, "Value 2"=0.0, "Command"=""}, {"Name"="", "Value 1"=20000.0, "Value 2"=0.0, "Command"=""}, {"Name"="", "Value 1"=30000.0, "Value 2"=0.0, "Command"=""}, {"Name"="", "Value 1"=50000.0, "Value 2"=0.0, "Command"=""}, {"Name"="", "Value 1"=100000.0, "Value 2"=0.0, "Command"=""}, {"Name"="", "Value 1"=200000.0, "Value 2"=0.0, "Command"=""}, {"Name"="", "Value 1"=300000.0, "Value 2"=0.0, "Command"=""}, {"Name"="", "Value 1"=500000.0, "Value 2"=0.0, "Command"=""}, {"Name"="", "Value 1"=1000000.0, "Value 2"=0.0, "Command"=""}, {"Name"="", "Value 1"=1080000.0, "Value 2"=0.0, "Command"=""}, {"Name"="", "Value 1"=2000000.0, "Value 2"=0.0, "Command"=""}, {"Name"="", "Value 1"=2700000.0, "Value 2"=0.0, "Command"=""}, {"Name"="", "Value 1"=3000000.0, "Value 2"=0.0, "Command"=""}, {"Name"="", "Value 1"=4500000.0, "Value 2"=0.0, "Command"=""}, {"Name"="", "Value 1"=5000000.0, "Value 2"=0.0, "Command"=""}, {"Name"="", "Value 1"=9000000.0, "Value 2"=0.0, "Command"=""}, {"Name"="", "Value 1"=10000000.0, "Value 2"=0.0, "Command"=""}, {"Name"="", "Value 1"=13500000.0, "Value 2"=0.0, "Command"=""}, {"Name"="", "Value 1"=18000000.0, "Value 2"=0.0, "Command"=""}, {"Name"="", "Value 1"=20000000.0, "Value 2"=0.0, "Command"=""}, {"Name"="", "Value 1"=30000000.0, "Value 2"=0.0, "Command"=""}, {"Name"="", "Value 1"=40000000.0, "Value 2"=0.0, "Command"=""}, {"Name"="", "Value 1"=2000.0, "Value 2"=0.0, "Command"=""}, {"Name"="", "Value 1"=1400000.0, "Value 2"=0.0, "Command"=""}, {"Name"="", "Value 1"=6000000.0, "Value 2"=0.0, "Command"=""}, {"Name"="", "Value 1"=9400000.0, "Value 2"=0.0, "Command"=""}, {"Name"="", "Value 1"=12000000.0, "Value 2"=0.0, "Command"=""}, {"Name"="", "Value 1"=14200000.0, "Value 2"=0.0, "Command"=""}, {"Name"="", "Value 1"=15000000.0, "Value 2"=0.0, "Command"=""}, {"Name"="", "Value 1"=17000000.0, "Value 2"=0.0, "Command"=""}, {"Name"="", "Value 1"=19000000.0, "Value 2"=0.0, "Command"=""}, {"Name"="", "Value 1"=23000000.0, "Value 2"=0.0, "Command"=""}, {"Name"="", "Value 1"=24000000.0, "Value 2"=0.0, "Command"=""}, {"Name"="", "Value 1"=28000000.0, "Value 2"=0.0, "Command"=""}, {"Name"="", "Value 1"=29000000.0, "Value 2"=0.0, "Command"=""}, {"Name"="", "Value 1"=38000000.0, "Value 2"=0.0, "Command"=""}, {"Name"="", "Value 1"=39000000.0, "Value 2"=0.0, "Command"=""}, {"Name"="", "Value 1"=45000000.0, "Value 2"=0.0, "Command"=""}, {"Name"="", "Value 1"=49000000.0, "Value 2"=0.0, "Command"=""}, {"Name"="", "Value 1"=56000000.0, "Value 2"=0.0, "Command"=""}, {"Name"="", "Value 1"=58000000.0, "Value 2"=0.0, "Command"=""}, {"Name"="", "Value 1"=60000000.0, "Value 2"=0.0, "Command"=""}, {"Name"="", "Value 1"=67000000.0, "Value 2"=0.0, "Command"=""}, {"Name"="", "Value 1"=68000000.0, "Value 2"=0.0, "Command"=""}, {"Name"="", "Value 1"=78000000.0, "Value 2"=0.0, "Command"=""}, {"Name"="", "Value 1"=80000000.0, "Value 2"=0.0, "Command"=""}, {"Name"="", "Value 1"=88000000.0, "Value 2"=0.0, "Command"=""}, {"Name"="", "Value 1"=89000000.0, "Value 2"=0.0, "Command"=""}, {"Name"="", "Value 1"=90000000.0, "Value 2"=0.0, "Command"=""}, {"Name"="", "Value 1"=98000000.0, "Value 2"=0.0, "Command"=""}, {"Name"="", "Value 1"=100000000.0, "Value 2"=0.0, "Command"=""}, {"Name"="", "Value 1"=112000000.0, "Value 2"=0.0, "Command"=""}, {"Name"="", "Value 1"=160000000.0, "Value 2"=0.0, "Command"=""}]}, {"Type"=2, "Name"="rsCmxpGprf_rngCMWSConnectorSet", "Entries"=[{"Name"="Global", "Value 1"=0.0, "Value 2"=0.0, "Command"="GLOB"}, {"Name"="List", "Value 1"=1.0, "Value 2"=0.0, "Command"="LIST"}]}, {"Type"=0, "Name"="rsCmxpGprf_rngListRange", "Entries"=[{"Name"="", "Value 1"=1.0, "Value 2"=2000.0, "Command"=""}]}, {"Type"=2, "Name"="rsCmxpGprf_rngCMWSConnSet", "Entries"=[{"Name"="Global", "Value 1"=0.0, "Value 2"=0.0, "Command"="GLOB"}, {"Name"="List", "Value 1"=1.0, "Value 2"=0.0, "Command"="LIST"}]}, {"Type"=0, "Name"="rsCmxpGprf_rngSequencerTriggerTimeout", "Entries"=[{"Name"="", "Value 1"=0.01, "Value 2"=300.0, "Command"=""}]}, {"Type"=2, "Name"="rsCmxpGprf_rngARBSamplesRange", "Entries"=[{"Name"="Full", "Value 1"=0.0, "Value 2"=0.0, "Command"="FULL"}, {"Name"="Sub", "Value 1"=1.0, "Value 2"=0.0, "Command"="SUB"}]}, {"Type"=0, "Name"="rsCmxpGprf_rngNRPMStatCount", "Entries"=[{"Name"="", "Value 1"=1.0, "Value 2"=1000.0, "Command"=""}]}, {"Type"=2, "Name"="rsCmxpGprf_rngStatus", "Entries"=[{"Name"="Off", "Value 1"=0.0, "Value 2"=0.0, "Command"="OFF"}, {"Name"="Run", "Value 1"=1.0, "Value 2"=0.0, "Command"="RUN"}, {"Name"="Ready", "Value 1"=2.0, "Value 2"=0.0, "Command"="RDY"}]}, {"Type"=2, "Name"="rsCmxpGprf_rngResourceStatus", "Entries"=[{"Name"="Queued", "Value 1"=0.0, "Value 2"=0.0, "Command"="QUE"}, {"Name"="Active", "Value 1"=1.0, "Value 2"=0.0, "Command"="ACT"}, {"Name"="Invalid", "Value 1"=2.0, "Value 2"=0.0, "Command"="INV"}]}, {"Type"=0, "Name"="rsCmxpGprf_rngNRPMMeasurementFrequency", "Entries"=[{"Name"="", "Value 1"=27500000000.0, "Value 2"=75000000000.0, "Command"=""}]}, {"Type"=2, "Name"="rsCmxpGprf_rngResultType", "Entries"=[{"Name"="Current", "Value 1"=0.0, "Value 2"=0.0, "Command"="CURR"}, {"Name"="Average", "Value 1"=1.0, "Value 2"=0.0, "Command"="AVER"}, {"Name"="Peak", "Value 1"=2.0, "Value 2"=0.0, "Command"="PEAK"}]}, {"Type"=2, "Name"="rsCmxpGprf_rngDetectorType", "Entries"=[{"Name"="RMS", "Value 1"=0.0, "Value 2"=0.0, "Command"="RMS"}, {"Name"="Minimum", "Value 1"=1.0, "Value 2"=0.0, "Command"="MIN"}, {"Name"="Maximum", "Value 1"=2.0, "Value 2"=0.0, "Command"="MAX"}]}, {"Type"=2, "Name"="rsCmxpGprf_rngPowerStatisticsTrace", "Entries"=[{"Name"="APD", "Value 1"=0.0, "Value 2"=0.0, "Command"="APD"}, {"Name"="CCDF", "Value 1"=1.0, "Value 2"=0.0, "Command"="CCDF"}]}, {"Type"=2, "Name"="rsCmxpGprf_rngIQSignal", "Entries"=[{"Name"="I", "Value 1"=0.0, "Value 2"=0.0, "Command"="I"}, {"Name"="Q", "Value 1"=1.0, "Value 2"=0.0, "Command"="Q"}]}, {"Type"=0, "Name"="rsCmxpGprf_rngSequencerFrequencyOffset", "Entries"=[{"Name"="", "Value 1"=-500000000.0, "Value 2"=500000000.0, "Command"=""}]}, {"Type"=0, "Name"="rsCmxpGprf_rngSequencerLevelRatio", "Entries"=[{"Name"="", "Value 1"=0.0, "Value 2"=100.0, "Command"=""}]}, {"Type"=0, "Name"="rsCmxpGprf_rngSequencerListCreate", "Entries"=[{"Name"="", "Value 1"=-inf, "Value 2"=inf, "Command"=""}]}, {"Type"=2, "Name"="rsCmxpGprf_rngListIncrement", "Entries"=[{"Name"="Dtime", "Value 1"=0.0, "Value 2"=0.0, "Command"="DTIM"}, {"Name"="Acycles", "Value 1"=1.0, "Value 2"=0.0, "Command"="ACYC"}, {"Name"="User", "Value 1"=2.0, "Value 2"=0.0, "Command"="USER"}, {"Name"="Measurement", "Value 1"=3.0, "Value 2"=0.0, "Command"="MEAS"}, {"Name"="Trigger", "Value 1"=4.0, "Value 2"=0.0, "Command"="TRIG"}]}, {"Type"=2, "Name"="rsCmxpGprf_rngListIncTransition", "Entries"=[{"Name"="Immediate", "Value 1"=0.0, "Value 2"=0.0, "Command"="IMM"}, {"Name"="Restart marker", "Value 1"=1.0, "Value 2"=0.0, "Command"="RMAR"}, {"Name"="Waveform marker 1", "Value 1"=2.0, "Value 2"=0.0, "Command"="WMA1"}, {"Name"="Waveform marker 2", "Value 1"=3.0, "Value 2"=0.0, "Command"="WMA2"}, {"Name"="Waveform marker 3", "Value 1"=4.0, "Value 2"=0.0, "Command"="WMA3"}, {"Name"="Waveform marker 4", "Value 1"=5.0, "Value 2"=0.0, "Command"="WMA4"}]}, {"Type"=0, "Name"="rsCmxpGprf_rngSequencerListTransitionTime", "Entries"=[{"Name"="", "Value 1"=0.0, "Value 2"=0.0005, "Command"=""}]}, {"Type"=0, "Name"="rsCmxpGprf_rngSequencerRestartMarkerDelay", "Entries"=[{"Name"="", "Value 1"=0.0, "Value 2"=0.1, "Command"=""}]}, {"Type"=0, "Name"="rsCmxpGprf_rngSequencerWaveformMarkerDelay", "Entries"=[{"Name"="", "Value 1"=0.0, "Value 2"=0.1, "Command"=""}]}, {"Type"=0, "Name"="rsCmxpGprf_rngSequenceRepetitionCount", "Entries"=[{"Name"="", "Value 1"=1.0, "Value 2"=1000.0, "Command"=""}]}, {"Type"=0, "Name"="rsCmxpGprf_rngBasebandTriggerDelay", "Entries"=[{"Name"="", "Value 1"=0.0, "Value 2"=100.0, "Command"=""}]}, {"Type"=0, "Name"="rsCmxpGprf_rngBasebandTriggerTimeout", "Entries"=[{"Name"="", "Value 1"=0.01, "Value 2"=300.0, "Command"=""}]}, {"Type"=0, "Name"="rsCmxpGprf_rngIQRecorderMeasurementTriggerPhaseChangeThreshold", "Entries"=[{"Name"="", "Value 1"=1.0, "Value 2"=180.0, "Command"=""}]}, {"Type"=0, "Name"="rsCmxpGprf_rngIQRecorderMeasurementTriggerPhaseChangeTime", "Entries"=[{"Name"="", "Value 1"=1e-06, "Value 2"=5e-05, "Command"=""}]}, {"Type"=2, "Name"="rsCmxpGprf_rngPowerMeasurementListTXIncrementMode", "Entries"=[{"Name"="Index Repetition", "Value 1"=0.0, "Value 2"=0.0, "Command"="IREP"}, {"Name"="List Entry", "Value 1"=1.0, "Value 2"=0.0, "Command"="LENT"}]}, {"Type"=2, "Name"="rsCmxpGprf_rngTargetSyncState", "Entries"=[{"Name"="Pending", "Value 1"=0.0, "Value 2"=0.0, "Command"="PEND"}, {"Name"="Adjusted", "Value 1"=1.0, "Value 2"=0.0, "Command"="ADJ"}]}] {"Type" items=["Range", "Coerced", "Discrete"]}
  in  "Attributes":T3[](array[typedef])=[{"Level"=1, "Class Only"=TRUE, "Identifier"="", "Descriptive Name"="Generator", "Data Type"=0, "Command"="", "Access"=0, "Range Table"="", "Read Callback"="", "Write Callback"="", "Supported Models"="", "Instrument Options"="", "Flags"=0, "Help"="Generator configuration."}, {"Level"=2, "Class Only"=FALSE, "Identifier"="RSCMXPGPRF_ATTR_GENERATOR_STATE", "Descriptive Name"="Generator State", "Data Type"=3, "Command"="SOUR:GPRF:GEN{instance}:STAT", "Access"=1, "Range Table"="", "Read Callback"="", "Write Callback"="", "Supported Models"="", "Instrument Options"="", "Flags"=0, "Help"="Turns the generator on or off.\n\nAvailable Repeated Capabilities:\ninstance: i0, i1, i2, i3, i4, i5, i6, i7, i8, i9, i10, i11, i12, i13, i14, i15, i16, i17, i18, i19, i20, i21, i22, i23, i24, i25, i26, i27, i28, i29, i30, i31, i32\r\n\nRemote-control command(s):\nSOURce:GPRF:GEN<i>:STATe"}, {"Level"=2, "Class Only"=FALSE, "Identifier"="RSCMXPGPRF_ATTR_QUERY_GENERATOR_STATE", "Descriptive Name"="Query Generator State", "Data Type"=0, "Command"="SOUR:GPRF:GEN{instance}:STAT?", "Access"=0, "Range Table"="rsCmxpGprf_rngGeneratorState", "Read Callback"="", "Write Callback"="", "Supported Models"="", "Instrument Options"="", "Flags"=0, "Help"="Queries generator state.\n\nAvailable Repeated Capabilities:\ninstance: i0, i1, i2, i3, i4, i5, i6, i7, i8, i9, i10, i11, i12, i13, i14, i15, i16, i17, i18, i19, i20, i21, i22, i23, i24, i25, i26, i27, i28, i29, i30, i31, i32\r\n\nRemote-control command(s):\nSOURce:GPRF:GEN<i>:STATe?"}, {"Level"=2, "Class Only"=FALSE, "Identifier"="RSCMXPGPRF_ATTR_GENERATOR_RELIABILITY", "Descriptive Name"="Generator Reliability", "Data Type"=2, "Command"="SOUR:GPRF:GEN{instance}:REL:ALL?", "Access"=0, "Range Table"="", "Read Callback"="", "Write Callback"="", "Supported Models"="", "Instrument Options"="", "Flags"=0, "Help"="Reports if and why there are problems generating the configured signal.\n\nAvailable Repeated Capabilities:\ninstance: i0, i1, i2, i3, i4, i5, i6, i7, i8, i9, i10, i11, i12, i13, i14, i15, i16, i17, i18, i19, i20, i21, i22, i23, i24, i25, i26, i27, i28, i29, i30, i31, i32\r\n\nRemote-control command(s):\nSOURce:GPRF:GEN<i>:RELiability:ALL?"}, {"Level"=2, "Class Only"=FALSE, "Identifier"="RSCMXPGPRF_ATTR_GENERATOR_STATUS_ALL", "Descriptive Name"="Generator Status All", "Data Type"=6, "Command"="SOUR:GPRF:GEN{instance}:STAT:ALL?", "Access"=0, "Range Table"="", "Read Callback"="", "Write Callback"="", "Supported Models"="", "Instrument Options"="", "Flags"=0, "Help"="Queries the states of the generator.\n\nWithout query parameters, the states are returned immediately.\n\nWith query parameters, the states are returned when the <TargetMainState> and the <TargetSyncState> are reached or when the <Timeout> expires.\n\nAvailable Repeated Capabilities:\ninstance: i0, i1, i2, i3, i4, i5, i6, i7, i8, i9, i10, i11, i12, i13, i14, i15, i16, i17, i18, i19, i20, i21, i22, i23, i24, i25, i26, i27, i28, i29, i30, i31, i32\r\n\nRemote-control command(s):\nSOURce:GPRF:GEN<i>:STATe:ALL?"}, {"Level"=2, "Class Only"=TRUE, "Identifier"="", "Descriptive Name"="Routing Settings", "Data Type"=0, "Command"="", "Access"=0, "Range Table"="", 
